vi "Keithley 2400 Setting Strings.vi"(8 "error in (no error)":errorcluster, 11 "Keithley 2400 Settings Ref":refnum<vi>) -> (0 "error out":errorcluster, 3 "Keithley 2400 Setting Strings":string[](array[string]))   [LabVIEW 2019]
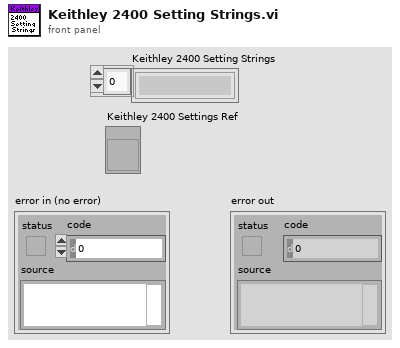
[diagram p1: front panel]
types:
  T1 = cluster{"Source Settings":enum32{"Voltage Source", "Current Source"}, "Current Compliance":dbl, "Voltage Compliance":dbl, "Use 4-Wire Sense":bool, "Voltage Auto Range":bool, "Voltage Manual Range":dbl, "Current Auto Range":bool, "Current Manual Range":dbl, "Measure Settings":cluster{"Voltage":bool, "Current":bool}, "Source Manual Range":dbl, "Source Auto Range":bool, "Reset Device":bool}
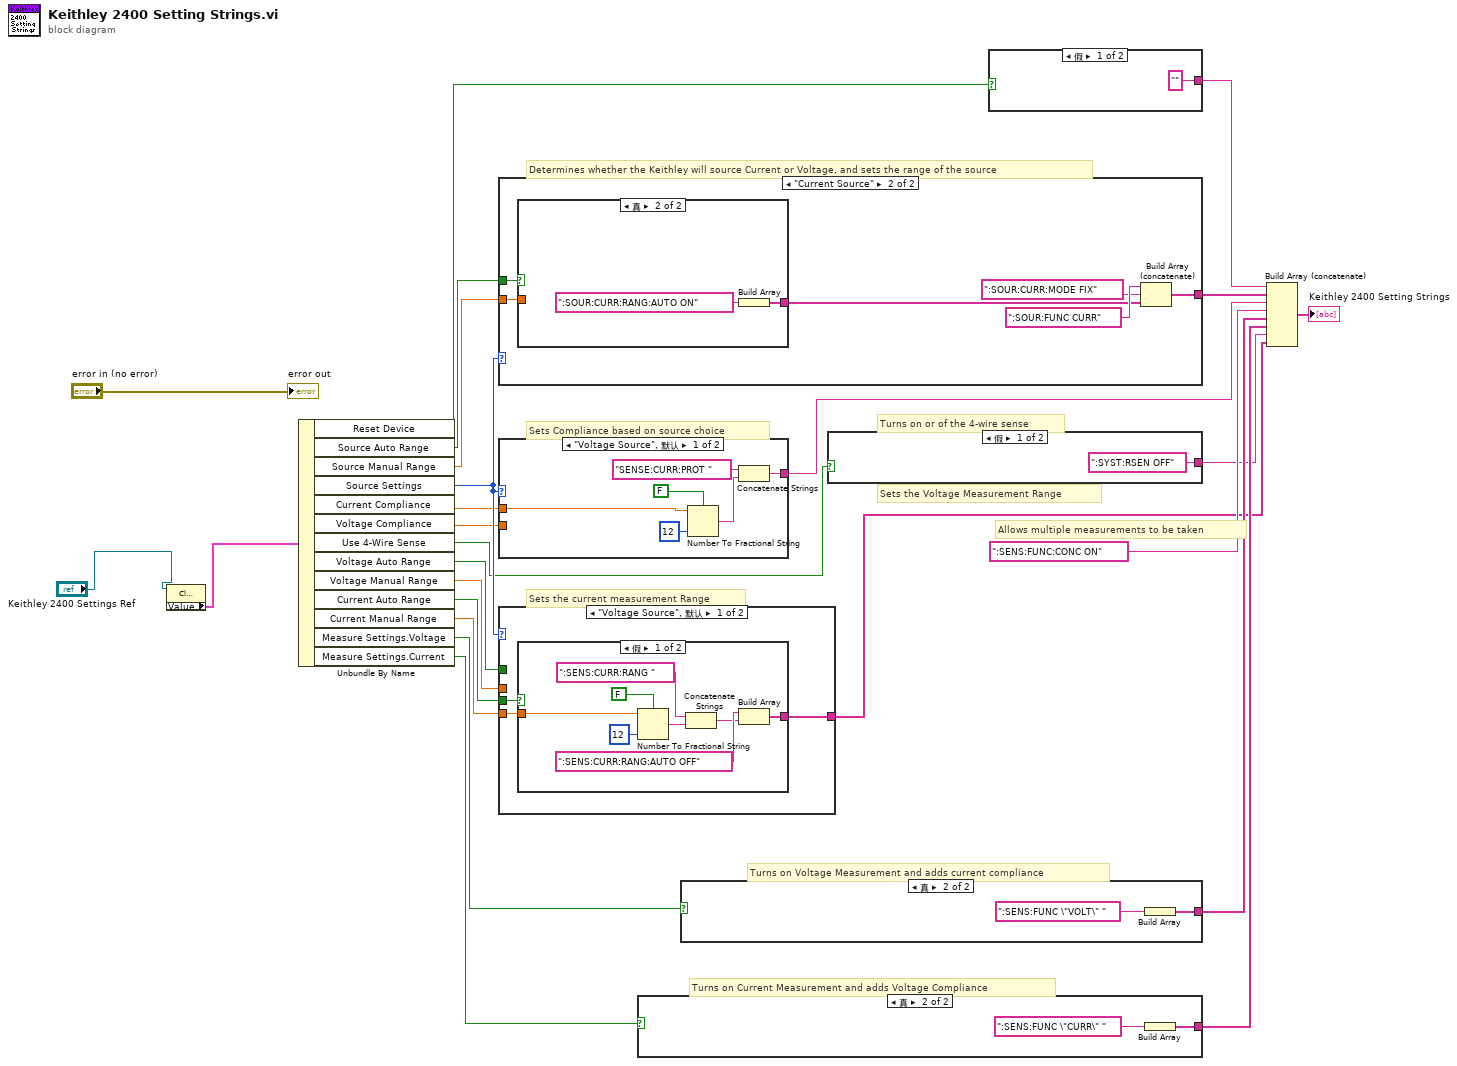
[diagram p0: block diagram]
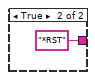
[diagram p2: hidden frame]
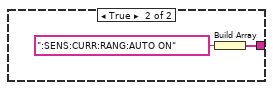
[diagram p3: hidden frame]
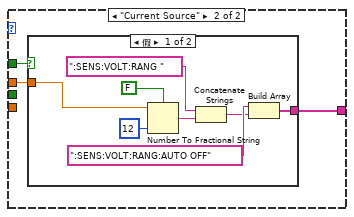
[diagram p4: hidden frame]
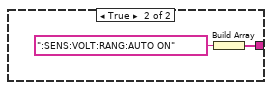
[diagram p5: hidden frame]
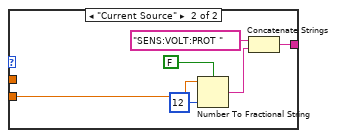
[diagram p6: hidden frame]
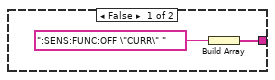
[diagram p7: hidden frame]
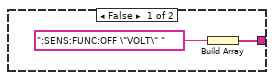
[diagram p8: hidden frame]
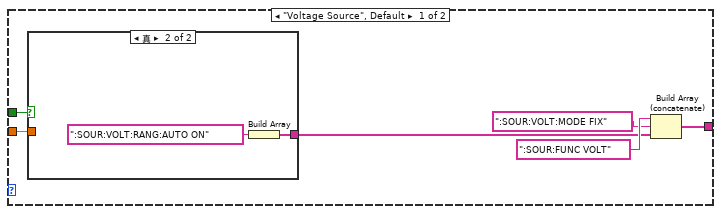
[diagram p9: hidden frame]
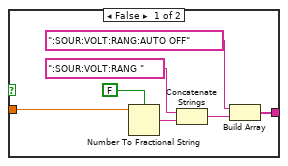
[diagram p10: hidden frame]
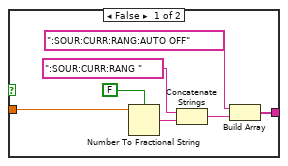
[diagram p11: hidden frame]
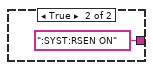
[diagram p12: hidden frame]
diagram:
  # "Sets Compliance based on source choice"
  # "Sets the current measurement Range"
  # "Sets the Voltage Measurement Range"
  # "Turns on or of the 4-wire sense"
  # "Allows multiple measurements to be taken"
  # "Turns on Current Measurement and adds Voltage Compliance"
  # "Turns on Voltage Measurement and adds current compliance"
  # "Determines whether the Keithley will source Current or Voltage, and sets the range of the source"
  n1 = property class="Clust (strict)"(reference="Keithley 2400 Settings Ref") -> ("Value"=w2:T1)  [unwired: 1 in, 2 out]
  n2 = Unbundle By Name(w2) -> ("Reset Device"=w24:bool, "Source Auto Range"=w12:bool, "Source Manual Range"=w11:dbl, "Source Settings"=w21:enum32{"Voltage Source", "Current Source"}, "Current Compliance"=w18:dbl, "Voltage Compliance"=w17:dbl, "Use 4-Wire Sense"=w15:bool, "Voltage Auto Range"=w10:bool, "Voltage Manual Range"=w9:dbl, "Current Auto Range"=w22:bool, "Current Manual Range"=w23:dbl, "Measure Settings.Voltage"=w14:bool, "Measure Settings.Current"=w13:bool)
  n3 = case shown="\"Current Source\"" w21 {
    tunnel: [w29 w44] -> w19
    tunnel: w12 -> [w28 w41]
    tunnel: w11 -> [w27 w43]
    frame "Voltage Source", Default {
      n4 = case shown="真" w28 {
        tunnel: w27 -> [w36 _]
        tunnel: [w32 w39] -> w26
        frame False {
          n5 = Number To Fractional String(use system decimal point (T)=FALSE, number=w36) -> (F-format string=w37:string)  [unwired: 2 in]
          n6 = Concatenate Strings(":SOUR:VOLT:RANG ", w37) -> (w33:string)
          n7 = Build Array(":SOUR:VOLT:RANG:AUTO OFF", w33) -> (w32:string[])
        }
        frame True {
          n8 = Build Array(":SOUR:VOLT:RANG:AUTO ON") -> (w39:string[])
        }
      }
      n9 = Build Array (concatenate)(":SOUR:FUNC VOLT", ":SOUR:VOLT:MODE FIX", w26) -> (w29:string[])
    }
    frame "Current Source" {
      n10 = case shown="真" w41 {
        tunnel: w43 -> [w51 _]
        tunnel: [w47 w54] -> w42
        frame False {
          n11 = Number To Fractional String(use system decimal point (T)=FALSE, number=w51) -> (F-format string=w52:string)  [unwired: 2 in]
          n12 = Concatenate Strings(":SOUR:CURR:RANG ", w52) -> (w48:string)
          n13 = Build Array(":SOUR:CURR:RANG:AUTO OFF", w48) -> (w47:string[])
        }
        frame True {
          n14 = Build Array(":SOUR:CURR:RANG:AUTO ON") -> (w54:string[])
        }
      }
      n15 = Build Array (concatenate)(":SOUR:FUNC CURR", ":SOUR:CURR:MODE FIX", w42) -> (w44:string[])
    }
  }
  n16 = case shown="\"Voltage Source\", 默认" w21 {
    tunnel: w17 -> [_ w64]
    tunnel: w18 -> [w58 _]
    tunnel: [w57 w63] -> w20
    frame "Voltage Source", Default {
      n17 = Number To Fractional String(use system decimal point (T)=FALSE, number=w58, precision (6)=i16 12) -> (F-format string=w60:string)  [unwired: 1 in]
      n18 = Concatenate Strings("SENSE:CURR:PROT ", w60) -> (w57:string)
    }
    frame "Current Source" {
      n19 = Number To Fractional String(use system decimal point (T)=FALSE, number=w64, precision (6)=i16 12) -> (F-format string=w66:string)  [unwired: 1 in]
      n20 = Concatenate Strings("SENS:VOLT:PROT ", w66) -> (w63:string)
    }
  }
  n21 = case shown="\"Voltage Source\", 默认" w21 {
    tunnel: [w68 w83] -> w4
    tunnel: w9 -> [_ w82]
    tunnel: w10 -> [_ w81]
    tunnel: w22 -> [w70 _]
    tunnel: w23 -> [w69 _]
    frame "Voltage Source", Default {
      n22 = case shown="假" w70 {
        tunnel: w69 -> [w76 _]
        tunnel: [w72 w79] -> w68
        frame False {
          n23 = Number To Fractional String(use system decimal point (T)=FALSE, number=w76, precision (6)=i16 12) -> (F-format string=w77:string)  [unwired: 1 in]
          n24 = Concatenate Strings(":SENS:CURR:RANG ", w77) -> (w73:string)
          n25 = Build Array(":SENS:CURR:RANG:AUTO OFF", w73) -> (w72:string[])
        }
        frame True {
          n26 = Build Array(":SENS:CURR:RANG:AUTO ON") -> (w79:string[])
        }
      }
    }
    frame "Current Source" {
      n27 = case shown="假" w81 {
        tunnel: w82 -> [w89 _]
        tunnel: [w85 w92] -> w83
        frame False {
          n28 = Number To Fractional String(use system decimal point (T)=FALSE, number=w89, precision (6)=i16 12) -> (F-format string=w90:string)  [unwired: 1 in]
          n29 = Concatenate Strings(":SENS:VOLT:RANG ", w90) -> (w86:string)
          n30 = Build Array(":SENS:VOLT:RANG:AUTO OFF", w86) -> (w85:string[])
        }
        frame True {
          n31 = Build Array(":SENS:VOLT:RANG:AUTO ON") -> (w92:string[])
        }
      }
    }
  }
  n32 = case shown="真" w13 {
    tunnel: [w94 w97] -> w6
    frame False {
      n33 = Build Array(":SENS:FUNC:OFF \"CURR\" ") -> (w94:string[])
    }
    frame True {
      n34 = Build Array(":SENS:FUNC \"CURR\" ") -> (w97:string[])
    }
  }
  n35 = case shown="真" w14 {
    tunnel: [w98 w100] -> w7
    frame False {
      n36 = Build Array(":SENS:FUNC:OFF \"VOLT\" ") -> (w98:string[])
    }
    frame True {
      n37 = Build Array(":SENS:FUNC \"VOLT\" ") -> (w100:string[])
    }
  }
  n38 = case shown="假" w15 {
    tunnel: [":SYST:RSEN OFF" ":SYST:RSEN ON"] -> w5
    frame False {
    }
    frame True {
    }
  }
  n39 = case shown="假" w24 {
    tunnel: ["" "*RST"] -> w25
    frame False {
    }
    frame True {
    }
  }
  n40 = Build Array (concatenate)(w25, w19, w20, ":SENS:FUNC:CONC ON", w7, w6, w5, w4) -> (→"Keithley 2400 Setting Strings":string[])
  "error out" <- "error in (no error)"
